vi "TriggerBdcst.vi"(8 "error in (no error)":errorcluster, 10 "Trigger":T1, 11 "Module":refnum<class "ModuleAdmin.lvclass">) -> (0 "error out":errorcluster, 3 "Module":refnum<class "ModuleAdmin.lvclass">)   [LabVIEW 2018, in "DigitizerPlugins.lvlib" / "DigitizerBase.lvclass"]
uses:
  DigitizerBase.lvclass
  <userlib>/NIST/ModuleAdminLib/ModuleAdmin/ModuleAdmin.lvclass
  Typedefs/Trigger.ctl
  Typedefs/TrigSource.ctl
  DigitizerShared/clEventType.ctl
  DigitizerShared/DigitizerShared.lvlib
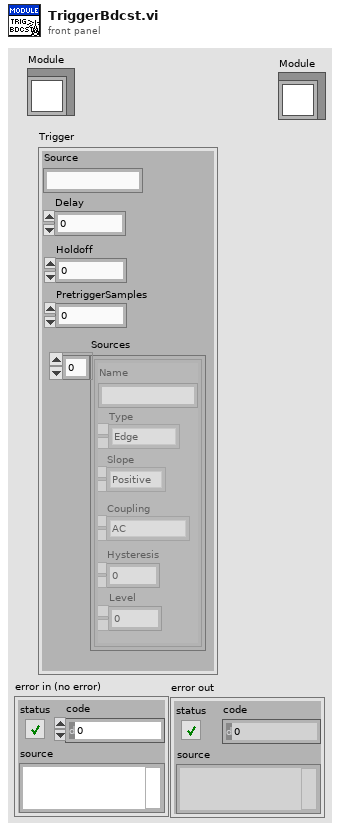
[diagram p1: front panel]
types:
  T1 = typedef "DigitizerPlugins.lvlib/DigitizerBase.lvclass/Trigger.ctl" = cluster{"Source":string, "Delay":dbl, "Holdoff":dbl, "PretriggerSamples":i32, "Sources":T2[]}
  T2 = typedef "DigitizerPlugins.lvlib/DigitizerBase.lvclass/TrigSource.ctl" = cluster{"Name":string, "Coupling":enum16{"AC", "DC", "HF Reject", "LF Reject", "Noise Reject"}, "Hysteresis":dbl, "Level":dbl, "Slope":enum16{"Positive", "Negative"}, "Type":enum16{"Edge", "Width", "Runt", "Glitch", "TV", "Window"}}
  T3 = typedef "DigitizerShared.lvlib/clEventType.ctl" = cluster{"ModuleID":i32, "Data":variant}
  T4 = typedef "DigitizerShared.lvlib/clBroadcastEvents.ctl" = cluster{"DidInit":refnum<user-event>, "StatusUpdate":refnum<user-event>, "ErrorReport":refnum<user-event>, "DidStop":refnum<user-event>, "PathToINI":refnum<user-event>, "Channels":refnum<user-event>, "Acq":refnum<user-event>, "Trigger":refnum<user-event>, "Waveforms":refnum<user-event>}
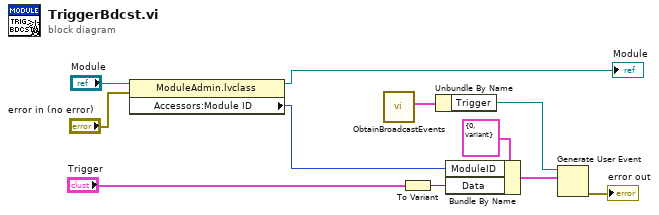
[diagram p0: block diagram]
diagram:
  n1 = property class="ModuleAdmin.lvclass"(reference="Module", error in="error in (no error)") -> (reference out=→"Module":refnum<class "ModuleAdmin.lvclass">, "Accessors:Module ID"=w4:i32)  [unwired: 1 out]
  n2 = call "ObtainBroadcastEvents.vi"() -> ("clDigitizerBdcstEvents"=w11:T4)  [unwired: 10 in, 1 out]
  n3 = To Variant(anything="Trigger") -> (Variant=w8:variant)
  n4 = Unbundle By Name(w11) -> ("Trigger"=w10:refnum<user-event>)
  n5 = Bundle By Name(cluster=T3 {"ModuleID"=0, "Data"=variant} ("clBroadcast"), "ModuleID"=w4, "Data"=w8) -> (w7:T3)
  n6 = Generate User Event(user event=w10, event data cluster=w7) -> (error out=→"error out":errorcluster)  [unwired: 2 in, 1 out]
